vi "Compute Motor Values.vi"(8 "Current Limit":dbl[unit]=1000.0, 9 "Effective Motor Voltage":dbl[unit]=12.0, 10 "Motor Model Values":T2 {"Breaker Size" format="%#_3p"; "Kv" format="%#_3p"; "R" format="%#_3p"; "Kt" format="%#_3p"}, 11 "motor speed (rpm)":dbl) -> (0 "chart values":T1, 1 "Power":dbl[unit] format="%#_3p", 2 "Motor Torque":dbl[unit] format="%#_3p", 3 "Current":dbl[unit] format="%#_3g")   [LabVIEW 2019]
uses:
  Modeling/Motor Operating Values.ctl
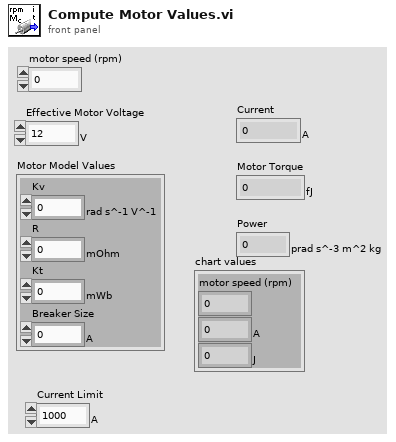
[diagram p1: front panel]
types:
  T1 = cluster{"motor speed (rpm)":dbl, dbl[unit], dbl[unit]}
  T2 = typedef "Motor Operating Values.ctl" = cluster{"Kv":dbl[unit], "R":dbl[unit], "Kt":dbl[unit], "Breaker Size":dbl[unit]}
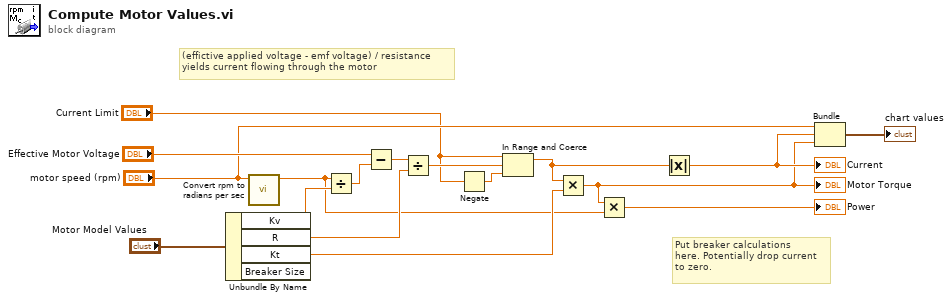
[diagram p0: block diagram]
diagram:
  # "Put breaker calculations\nhere. Potentially drop current\nto zero."
  # "(effictive applied voltage - emf voltage) / resistance\nyields current flowing through the motor"
  n1 = Unbundle By Name("Motor Model Values") -> ("Kv"=w15:dbl[unit], "R"=w16:dbl[unit], "Kt"=w17:dbl[unit])  [unwired: 1 out]
  n2 = call "Convert rpm to radians per sec.vi"("motor speed (rpm)"="motor speed (rpm)") -> ("speed rps"=w13:dbl[unit])  [unwired: 10 in]
  n3 = Divide(x=w13, y=w15) -> (x/y=w11:dbl[unit])
  n4 = Subtract(x="Effective Motor Voltage", y=w11) -> (x-y=w12:dbl[unit])
  n5 = Divide(x=w12, y=w16) -> (x/y=w4:dbl[unit])
  n6 = Negate(x="Current Limit") -> (-x=w2:dbl[unit])
  n7 = In Range and Coerce(upper limit="Current Limit", x=w4, lower limit=w2) -> (coerced(x)=w3:dbl[unit])  [unwired: 1 out]
  n8 = Multiply(x=w3, y=w17) -> (x*y=w7:dbl[unit])
  "Motor Torque" <- w7
  n9 = Multiply(x=w7, y=w13) -> (x*y=→"Power":dbl[unit])
  n10 = Absolute Value(x=w3) -> (abs(x)=w8:dbl[unit])
  "Current" <- w8
  n11 = Bundle("motor speed (rpm)"="motor speed (rpm)", w8, w7) -> (→"chart values":T1)  [unwired: 1 in]
